vi "PreOpenDevice.vi"(6 "aotuConn?":bool, 9 "Index":u32, 10 "type":u16(ring)=2 items=["USB-CAN"=2, "USB-CAN2.0"=3], 11 "param":T1[](array[typedef]) {"ACR0" format="%x"}) -> (1 "Channels":u32[](array[numeric]), 2 "DevIndex":u32, 3 "param out":T1[](array[typedef]) {"ACR0" format="%x"})   [LabVIEW 2011]
uses:
  Param.ctl
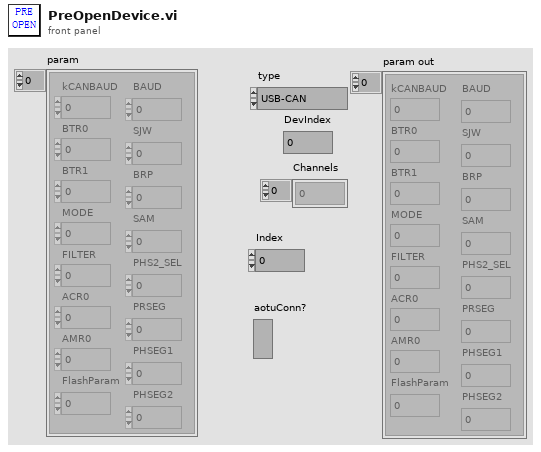
[diagram p1: front panel]
types:
  T1 = typedef "Param.ctl" = cluster{"kCANBAUD":u8, "BTR0":u8, "BTR1":u8, "MODE":u8, "FILTER":u8, "ACR0":u32, "AMR0":u32, "FlashParam":u32, "BAUD":u32, "SJW":u8, "BRP":u8, "SAM":u8, "PHS2_SEL":u8, "PRSEG":u8, "PHSEG1":u8, "PHSEG2":u8}
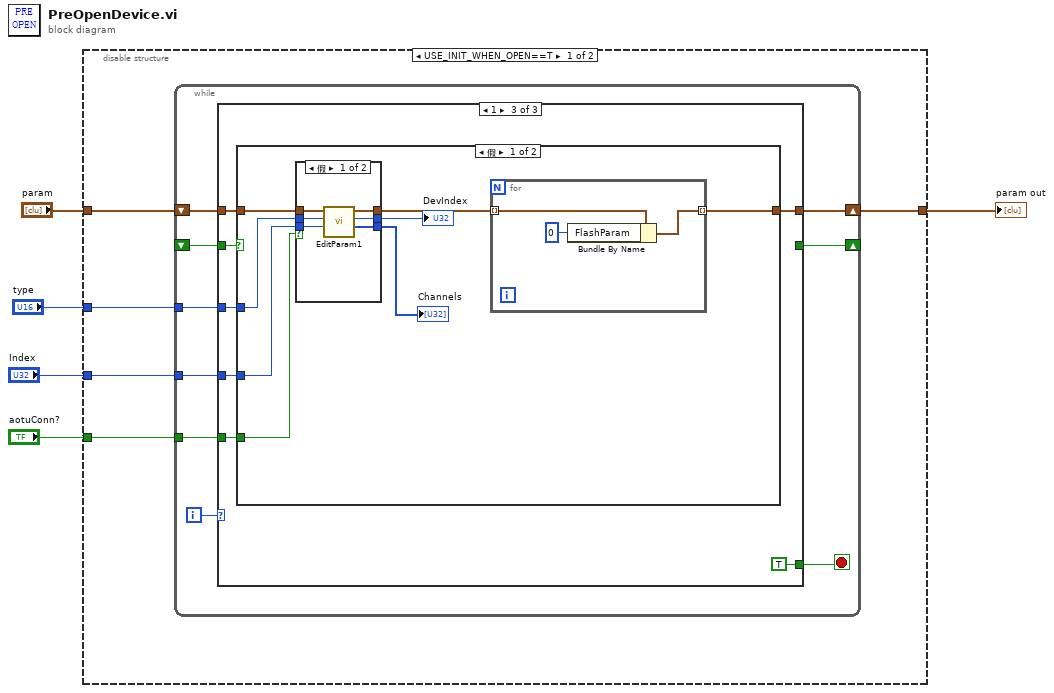
[diagram p0: block diagram]
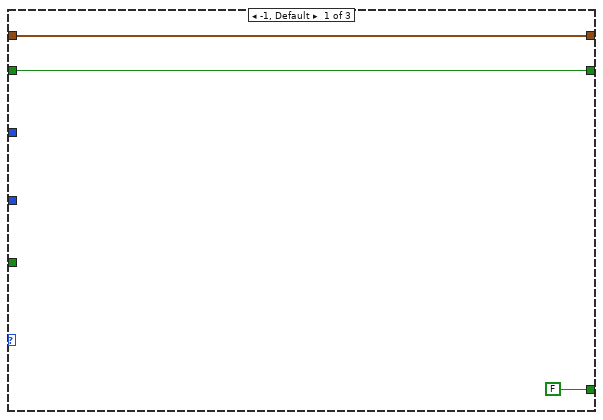
[diagram p2: hidden frame]
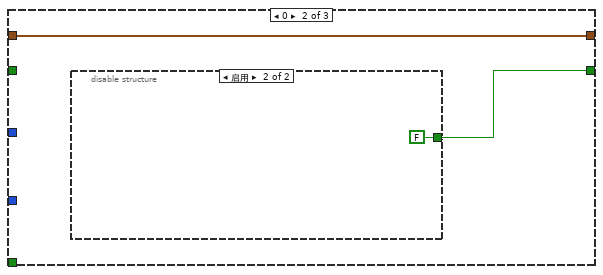
[diagram p3: hidden frame]
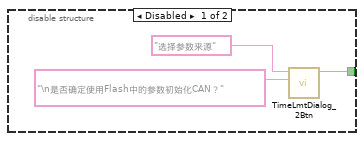
[diagram p4: hidden frame]
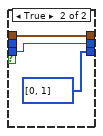
[diagram p5: hidden frame]
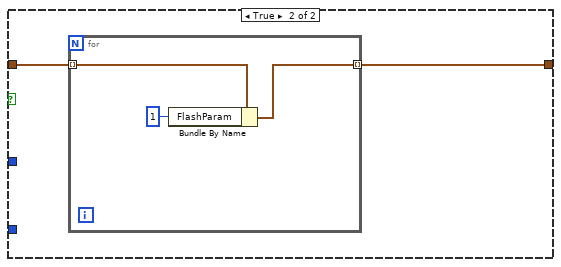
[diagram p6: hidden frame]
diagram:
  n1 = disable-structure shown="USE_INIT_WHEN_OPEN==T" {
    disable-tunnel: "param" -> [w10 w61]
    disable-tunnel: [w9 w61] -> w3
    disable-tunnel: "type" -> [w8 _]
    disable-tunnel: "Index" -> [w7 _]
    disable-tunnel: "aotuConn?" -> [w6 _]
    frame condition #0 (active) {
      n2 = while {
        shift-right: [w17] -> w9
        shift-left: w10 -> [w18]
        shift-right: [w15] -> _
        shift-left: _ -> [w14]
        tunnel: w8 -> [w13]
        tunnel: w7 -> [w12]
        tunnel: w6 -> [w11]
        i -> [w19]
        stop <- w16 stop-if-true
        n3 = case shown="1" w19 {
          tunnel: w18 -> [w22 w24 w34]
          tunnel: [w22 w24 w33] -> w17
          tunnel: [FALSE _ TRUE] -> w16
          tunnel: [w20 w23 _] -> w15
          tunnel: w14 -> [w20 _ w35]
          tunnel: w13 -> [_ _ w32]
          tunnel: w12 -> [_ _ w30]
          tunnel: w11 -> [_ _ w29]
          frame -1, Default {
          }
          frame 0 {
            n4 = disable-structure shown="启用" {
              disable-tunnel: [w25 FALSE ("OK?")] -> w23
              frame Disabled {
                n5 = call "TimeLmtDialog_2Btn.vi"("Infoin"="\n是否确定使用Flash中的参数初始化CAN？", "title"="选择参数来源") -> ("OK?"=w25:bool)  [unwired: 9 in]
              }
              frame Enabled {
              }
            }
          }
          frame 1 {
            n6 = case shown="假" w35 {
              tunnel: w34 -> [w43 w57]
              tunnel: [w41 w56] -> w33
              tunnel: w32 -> [w40 _]
              tunnel: w30 -> [w37 _]
              tunnel: w29 -> [w36 _]
              frame False {
                n7 = case shown="假" w36 {
                  tunnel: w43 -> [w49 w50]
                  tunnel: [w48 w50] -> w42
                  tunnel: w40 -> [w47 _]
                  tunnel: [w46 w51] -> w39
                  tunnel: [w45 u32[] [0, 1] ("Channels")] -> w38
                  tunnel: w37 -> [w44 w51]
                  frame False {
                    n8 = call "EditParam1.vi"("Index"=w44, "type"=w47, "param"=w49) -> ("Channels"=w45:u32[], "DevIndex"=w46:u32, "param out"=w48:T1[])  [unwired: 6 in]
                  }
                  frame True {
                  }
                }
                "DevIndex" <- w39
                "Channels" <- w38
                n9 = for {
                  tunnel: w42 -> [w55] mode=indexing
                  tunnel: [w54] -> w41 mode=indexing
                  n10 = Bundle By Name(cluster=w55, "FlashParam"=u32 0) -> (w54:T1)
                }
              }
              frame True {
                n11 = for {
                  tunnel: w57 -> [w60] mode=indexing
                  tunnel: [w58] -> w56 mode=indexing
                  n12 = Bundle By Name(cluster=w60, "FlashParam"=u32 1) -> (w58:T1)
                }
              }
            }
          }
        }
      }
    }
    frame condition #1 {
    }
  }
  "param out" <- w3
